vi "ReadReference.vi"(11 "DataValueRef":refnum<data-value>) -> (1 "ActiveChatId":i32, 2 "Token":string, 3 "FPFARef":refnum<k20>)   [LabVIEW 2015]
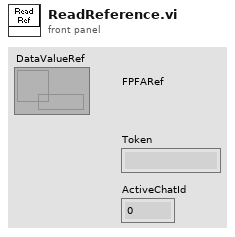
[diagram p1: front panel]
types:
  T1 = cluster{"FPGA VI Ref":refnum<k20>, "Token":string, "ActiveChatId":i32}
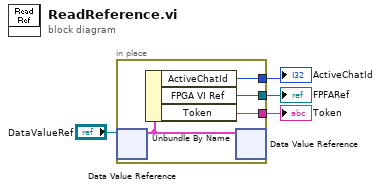
[diagram p0: block diagram]
diagram:
  n1 = in-place {
    in-place-border: [w7] -> w3
    in-place-border: [w6] -> w4
    in-place-border: [w5] -> w1
    n2 = in-place-dvr #1("DataValueRef") -> (w8:T1)  [unwired: 1 out]
    n3 = Unbundle By Name(w8) -> ("ActiveChatId"=w5:i32, "FPGA VI Ref"=w7:refnum<k20>, "Token"=w6:string)
    n4 = in-place-dvr #1(w8) -> ()  [unwired: 2 out]
  }
  "Token" <- w4
  "FPFARef" <- w3
  "ActiveChatId" <- w1
